vi "gyroscope mecanum thing.vi"(9 "Direction":dbl, 10 "gyroscope position":dbl, 11 "Target Position":dbl) -> (0 "backRight":dbl, 1 "backLeft":dbl, 2 "frontRight":dbl, 3 "frontLeft":dbl)   [LabVIEW 2019]
uses:
  <vilib>/Rock Robotics/Network Tables/NT Read Number.vi
panel:
  out "Numeric":dbl
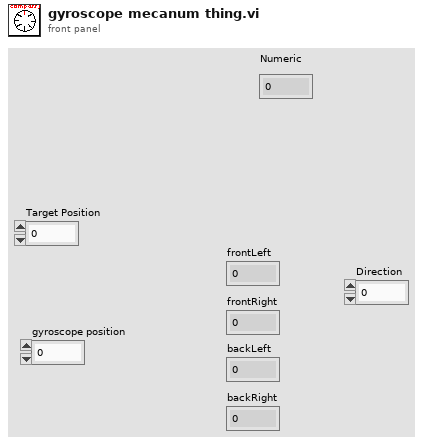
[diagram p1: front panel]
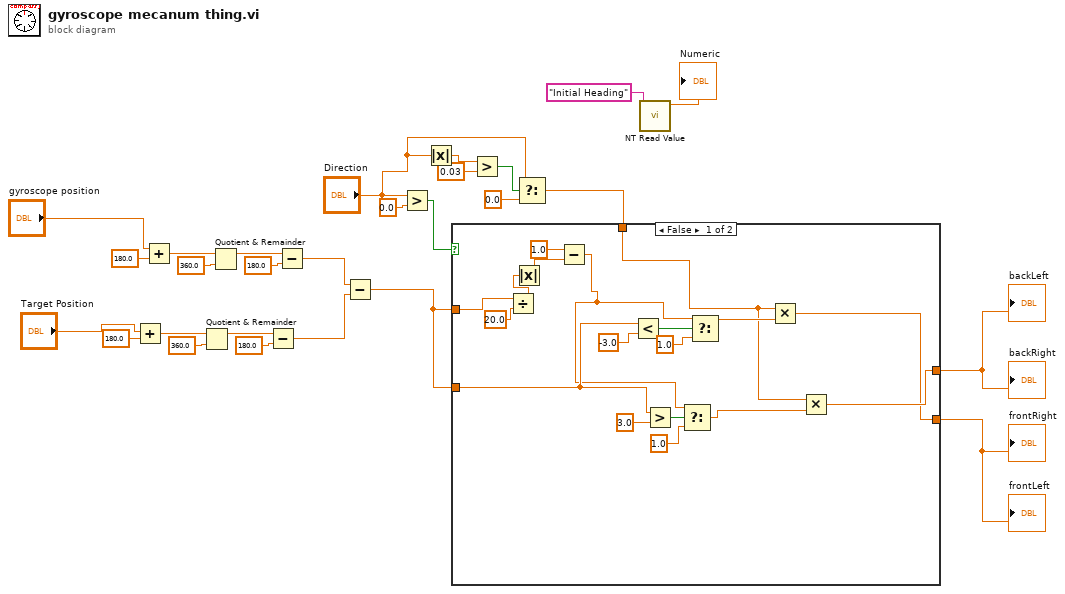
[diagram p0: block diagram]
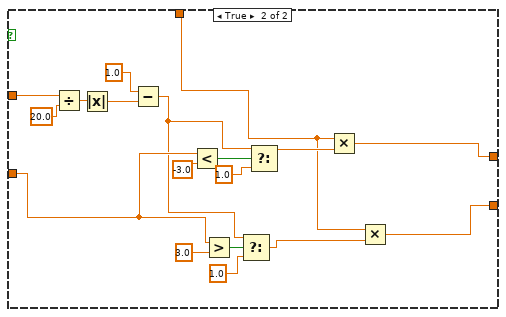
[diagram p2: hidden frame]
diagram:
  n1 = Add(x="Target Position", y=180.0) -> (x+y=w16:dbl)
  n2 = Add(x="gyroscope position", y=180.0) -> (x+y=w22:dbl)
  n3 = Quotient & Remainder(x=w16, y=360.0) -> (x-y*floor(x/y)=w14:dbl)  [unwired: 1 out]
  n4 = Quotient & Remainder(x=w22, y=360.0) -> (x-y*floor(x/y)=w20:dbl)  [unwired: 1 out]
  n5 = Subtract(x=w14, y=180.0) -> (x-y=w10:dbl)
  n6 = Subtract(x=w20, y=180.0) -> (x-y=w11:dbl)
  n7 = Subtract(x=w11, y=w10) -> (x-y=w1:dbl)
  n8 = Greater?(x="Direction", y=0.0) -> (0:w25:bool)
  n9 = Absolute Value(x="Direction") -> (abs(x)=w8:dbl)
  n10 = Greater?(x=w8, y=0.03) -> (0:w6:bool)
  n11 = Select(t="Direction", s=w6, f=0.0) -> (s? t:f=w4:dbl)
  n12 = case shown="False" w25 {
    tunnel: [w35 w53] -> w26
    tunnel: [w34 w52] -> w27
    tunnel: w4 -> [w36 w55]
    tunnel: w1 -> [w41 w54]
    tunnel: w1 -> [w33 w50]
    frame False {
      n13 = Divide(x=w33, y=20.0) -> (x/y=w28:dbl)
      n14 = Absolute Value(x=w28) -> (abs(x)=w29:dbl)
      n15 = Subtract(x=1.0, y=w29) -> (x-y=w30:dbl)
      n16 = Less?(x=w41, y=-3.0) -> (x < y?=w43:bool)
      n17 = Greater?(x=w41, y=3.0) -> (0:w45:bool)
      n18 = Select(t=w30, s=w45, f=1.0) -> (s? t:f=w39:dbl)
      n19 = Select(t=w30, s=w43, f=1.0) -> (s? t:f=w40:dbl)
      n20 = Multiply(x=w36, y=w40) -> (x*y=w34:dbl)
      n21 = Multiply(x=w36, y=w39) -> (x*y=w35:dbl)
    }
    frame True {
      n22 = Divide(x=w50, y=20.0) -> (x/y=w47:dbl)
      n23 = Absolute Value(x=w47) -> (abs(x)=w46:dbl)
      n24 = Subtract(x=1.0, y=w46) -> (x-y=w48:dbl)
      n25 = Less?(x=w54, y=-3.0) -> (x < y?=w61:bool)
      n26 = Greater?(x=w54, y=3.0) -> (0:w63:bool)
      n27 = Select(t=w48, s=w63, f=1.0) -> (s? t:f=w58:dbl)
      n28 = Select(t=w48, s=w61, f=1.0) -> (s? t:f=w59:dbl)
      n29 = Multiply(x=w55, y=w59) -> (x*y=w53:dbl)
      n30 = Multiply(x=w55, y=w58) -> (x*y=w52:dbl)
    }
  }
  "frontLeft" <- w27
  "frontRight" <- w27
  "backLeft" <- w26
  "backRight" <- w26
  n31 = call-poly <vilib>:"NT Read Value.vi"("Name"="Initial Heading") -> ("Numeric"=→"Numeric":dbl)  [unwired: 9 in, 1 out]
